vi "DIAdem Run Script.vi"(6 "asynchronous? (F)":bool, 8 "error in (no error)":errorcluster, 10 "script file":path, 11 "DIAdem Reference":T1) -> (0 "error out":errorcluster, 3 "DIAdem Reference":T1)   [LabVIEW 2017]
doc: "This VI runs the specified script in DIAdem. Specify the file name and directory of the script to run."
uses:
  <vilib>/ExportToExcel/DIAdem Reference.ctl
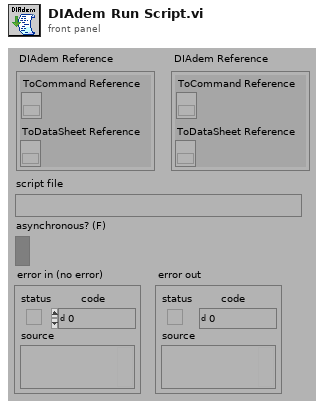
[diagram p1: front panel]
types:
  T1 = typedef "DIAdem Reference.ctl" = cluster{"ToCommand Reference":refnum<k7>, "ToDataSheet Reference":refnum<k7>}
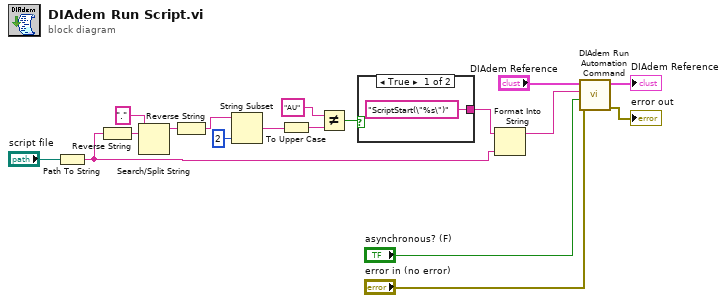
[diagram p0: block diagram]
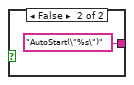
[diagram p2: hidden frame]
diagram:
  n1 = Path To String(path="script file") -> (string=w4:string)
  n2 = Reverse String(1:w4) -> (0:w10:string)
  n3 = Search/Split String(string=w10, search string/char (-)="." ("search char (-)")) -> (substring before match=w9:string)  [unwired: 1 in, 2 out]
  n4 = Reverse String(1:w9) -> (0:w2:string)
  n5 = String Subset(string=w2, length (rest)=2 ("length (rest)")) -> (substring=w3:string)  [unwired: 1 in]
  n6 = To Upper Case(1:w3) -> (0:w8:string)
  n7 = Not Equal?(x="AU" ("Substring"), y=w8) -> (x != y?=w5:bool)
  n8 = case shown="True" w5 {
    tunnel: ["ScriptStart(\"%s\")" ("Substring") "AutoStart(\"%s\")" ("Substring")] -> w13
    frame True {
    }
    frame False {
    }
  }
  n9 = Format Into String(format string=w13, w4) -> (resulting string=w12:string)  [unwired: 2 in, 1 out]
  n10 = call <vilib>:"DIAdem Run Automation Command.vi"("error in (no error)"="error in (no error)", "asynchronous? (F)"="asynchronous? (F)", "command"=w12, "DIAdem Reference"="DIAdem Reference") -> ("error out"=→"error out":errorcluster, "DIAdem Reference"=→"DIAdem Reference":T1)  [unwired: 6 in]
